vi "ConnectionHelper.vi"(7 "Reference":T1, 8 "ErrorIn":errorcluster, 11 "InCluster":T3) -> (0 "ErrorOut":errorcluster, 3 "OutCluster":T2, 5 "ReferenceOut":T1)   [LabVIEW 2022 SP3]
uses:
  C:/Users/Robots/Documents/robocadSimLV/assemblies/LibraryForLabVIEW.dll
  assemblies/LibraryForLabVIEW.dll
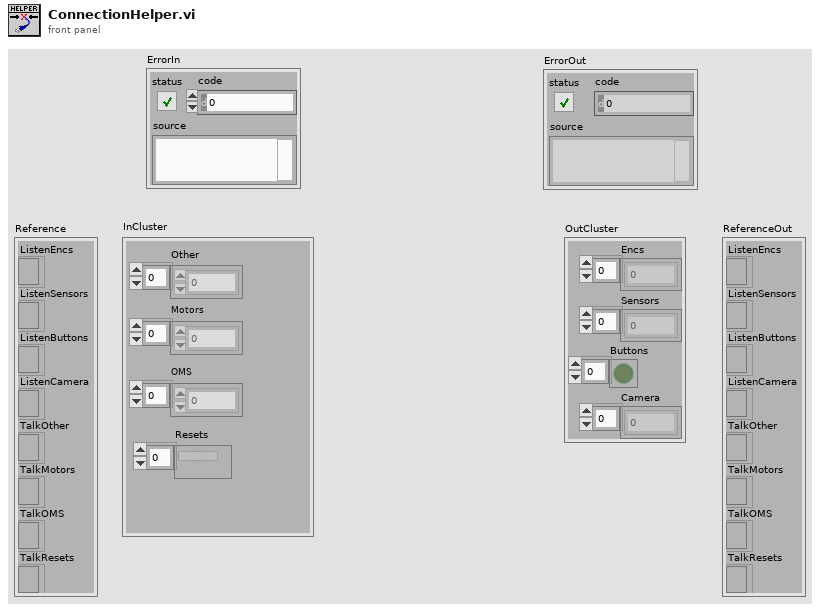
[diagram p1: front panel]
types:
  T1 = cluster{"ListenEncs":refnum<k24>, "ListenSensors":refnum<k24>, "ListenButtons":refnum<k24>, "ListenCamera":refnum<k24>, "TalkOther":refnum<k24>, "TalkMotors":refnum<k24>, "TalkOMS":refnum<k24>, "TalkResets":refnum<k24>}
  T2 = cluster{"Encs":dbl[], "Sensors":dbl[], "Buttons":bool[], "Camera":u8[]}
  T3 = cluster{"Other":dbl[], "Motors":dbl[], "OMS":dbl[], "Resets":bool[]}
  T4 = cluster{"Array":dbl[], "Array":dbl[], "Array":bool[], "OutBytes":u8[]}
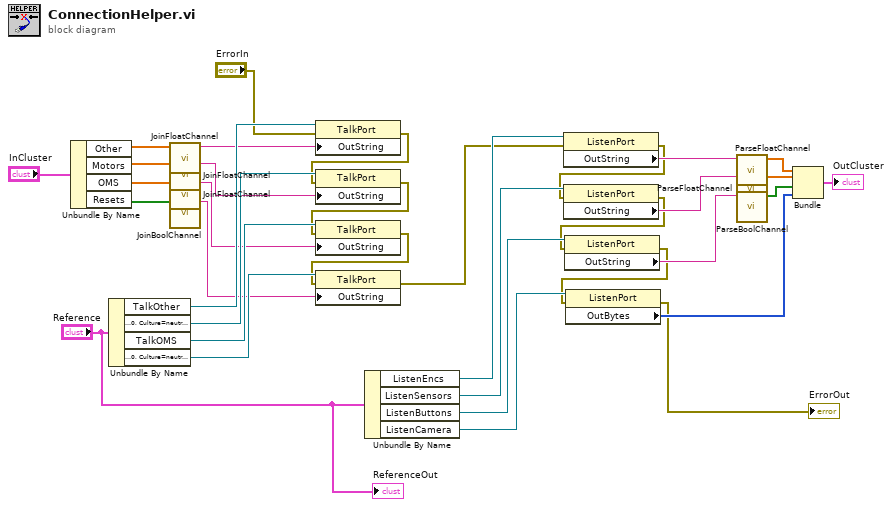
[diagram p0: block diagram]
diagram:
  n1 = Unbundle By Name("InCluster") -> ("Other"=w34:dbl[], "Motors"=w33:dbl[], "OMS"=w32:dbl[], "Resets"=w31:bool[])
  n2 = Unbundle By Name("Reference") -> ("TalkOther"=w27:refnum<k24>, "TalkMotors"=w25:refnum<k24>, "TalkOMS"=w23:refnum<k24>, "TalkResets"=w21:refnum<k24>)
  n3 = call "JoinFloatChannel.vi"("Array"=w34) -> ("String"=w26:string)  [unwired: 10 in]
  n4 = call "JoinFloatChannel.vi"("Array"=w33) -> ("String"=w24:string)  [unwired: 10 in]
  n5 = call "JoinFloatChannel.vi"("Array"=w32) -> ("String"=w22:string)  [unwired: 10 in]
  n6 = call "JoinBoolChannel.vi"("Array"=w31) -> ("String"=w20:string)  [unwired: 10 in]
  n7 = property class="TalkPort"(reference=w27, error in="ErrorIn", "OutString"=w26) -> (error out=w18:errorcluster)  [unwired: 1 out]
  n8 = property class="TalkPort"(reference=w25, error in=w18, "OutString"=w24) -> (error out=w17:errorcluster)  [unwired: 1 out]
  n9 = property class="TalkPort"(reference=w23, error in=w17, "OutString"=w22) -> (error out=w16:errorcluster)  [unwired: 1 out]
  n10 = property class="TalkPort"(reference=w21, error in=w16, "OutString"=w20) -> (error out=w6:errorcluster)  [unwired: 1 out]
  n11 = Unbundle By Name("Reference") -> ("ListenEncs"=w15:refnum<k24>, "ListenSensors"=w13:refnum<k24>, "ListenButtons"=w11:refnum<k24>, "ListenCamera"=w9:refnum<k24>)
  n12 = property class="ListenPort"(reference=w15, error in=w6) -> (error out=w5:errorcluster, "OutString"=w14:string)  [unwired: 1 out]
  n13 = property class="ListenPort"(reference=w13, error in=w5) -> (error out=w4:errorcluster, "OutString"=w12:string)  [unwired: 1 out]
  n14 = property class="ListenPort"(reference=w11, error in=w4) -> (error out=w3:errorcluster, "OutString"=w10:string)  [unwired: 1 out]
  n15 = property class="ListenPort"(reference=w9, error in=w3) -> (error out=→"ErrorOut":errorcluster, "OutBytes"=w8:u8[])  [unwired: 1 out]
  n16 = call "ParseFloatChannel.vi"("Input"=w14) -> ("Array"=w30:dbl[])  [unwired: 10 in]
  n17 = call "ParseFloatChannel.vi"("Input"=w12) -> ("Array"=w29:dbl[])  [unwired: 10 in]
  n18 = call "ParseBoolChannel.vi"("Input"=w10) -> ("Array"=w28:bool[])  [unwired: 10 in]
  n19 = Bundle("Array"=w30, "Array"=w29, "Array"=w28, "OutBytes"=w8) -> (→"OutCluster":T4)  [unwired: 1 in]
  "ReferenceOut" <- "Reference"
